vi "template_Job_Static_VI_Reference.vi"() -> ()   [LabVIEW 2013]
uses:
  Job/Job.lvclass
  Job/Job.lvclass/Job.ctl
  Job/Read Abort Notifier.vi
  <vilib>/Utility/error.llb/Error Cluster From Error Code.vi
panel:
  out "Job out":refnum<class "Job.lvclass">
  out "error out":errorcluster
  in  "Job":refnum<class "Job.lvclass">
  out "stdout":string
  in  "stdin":string
  # "All Controls and Indicators are optional and do not need to be connected to the ConPane\n\n\n-- \"Job\" class input allows to monitor the Abort notifications from scheduler.\n-- \"Job\" class output allows to insert key-value pairs into data map.\n-- stdin allows to pass in commands into the job\n-- stdout allows to send back a response to the scheduler after execution completes\n-- error output terminal returns the exception code to the scheduler\n-- stdin and stdout are default labels. If they are to be named differently, one must configure the constructor node declaring the Static VI refnum."
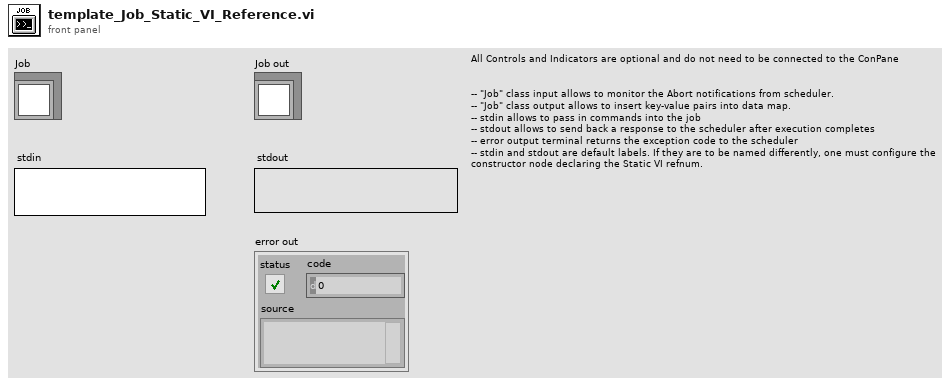
[diagram p1: front panel]
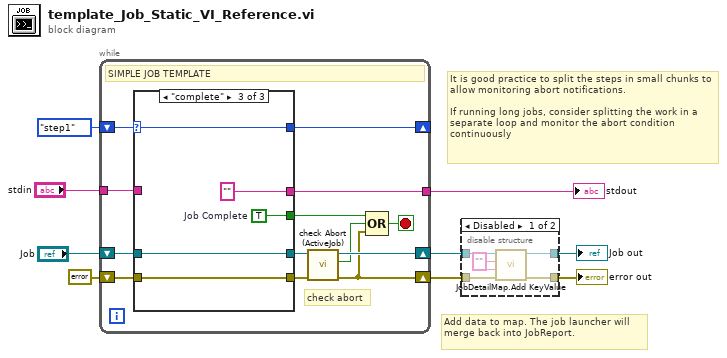
[diagram p0: block diagram]
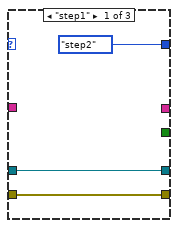
[diagram p3: hidden frame]
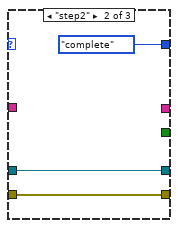
[diagram p4: hidden frame]
diagram:
  # "It is good practice to split the steps in small chunks to allow monitoring abort notifications.\n\nIf running long jobs, consider splitting the work in a separate loop and monitor the abort condition continuously"
  # "Add data to map. The job launcher will merge back into JobReport."
  n1 = while {
    tunnel: [w10] -> w4
    shift-right: [w20] -> w5
    shift-left: errorcluster {"status"=FALSE, "code"=0, "source"=""} ("error out") -> [w15]
    shift-right: [w21] -> w6
    shift-left: "Job" -> [w16]
    tunnel: "stdin" -> [w13]
    shift-right: [w11] -> _
    shift-left: enum16{"step1", "step2", "complete"}."step1" -> [w12]
    stop <- w22 stop-if-true
    # "check abort"
    # "SIMPLE JOB TEMPLATE"
    n2 = case shown="\"complete\"" w12 {
      selector: w12 -> [_ _ w30]
      tunnel: [_ _ w33] -> w18
      tunnel: [w25 w28 w32] -> w17
      tunnel: w16 -> [w25 w28 w32]
      tunnel: w15 -> [w24 w27 w31]
      tunnel: [w24 w27 w31] -> w14
      tunnel: w13 -> [_ _ _]
      tunnel: [enum16{"step1", "step2", "complete"}."step2" enum16{"step1", "step2", "complete"}."complete" w30] -> w11
      tunnel: [_ _ ""] -> w10
      frame "step1" {
      }
      frame "step2" {
      }
      frame "complete" {
        w33 = TRUE  # Job Complete
      }
    }
    n3 = call "check Abort (ActiveJob).vi"("error in (no error)"=w14, "Job in"=w17) -> ("error out"=w20:errorcluster, "Abort"=w19:bool, "Job out"=w21:refnum<class "Job.lvclass">)  [unwired: 6 in, 1 out]
    n4 = Compound Arithmetic op=OR(w18, w19, w20) -> (w22:bool)
  }
  "stdout" <- w4
  n5 = disable-structure shown="Disabled" {
    disable-tunnel: [w38 w40] -> w9
    disable-tunnel: [w37 w39] -> w8
    disable-tunnel: w6 -> [w36 w40]
    disable-tunnel: w5 -> [w35 w39]
    frame Disabled {
      w34 = "" ("Key")
      n6 = call "JobDetailMap.Add KeyValue.vi"("error in (no error)"=w35, "Value"=w34, "Key"=w34, "Job in"=w36) -> ("error out"=w37:errorcluster, "Job out"=w38:refnum<class "Job.lvclass">)  [unwired: 6 in]
    }
    frame Enabled {
    }
  }
  "error out" <- w8
  "Job out" <- w9
